vi "hse-application_SetApplicationVersion.vi"(8 "error in":errorcluster, 10 "Application Version History":string, 11 "Application Version Number":string) -> (0 "error out":errorcluster)   [LabVIEW 2014, in "hse-application.lvclass"]
doc: "Stores the version number of the application for later usage (display, logging, ...).\n\n\n\n____\nHAMPEL SOFTWARE ENGINEERING v0.12.0 (2018-09-13 18:21)"
uses:
  hse-application.lvclass
  hse-application.lvclass/hse-application.ctl
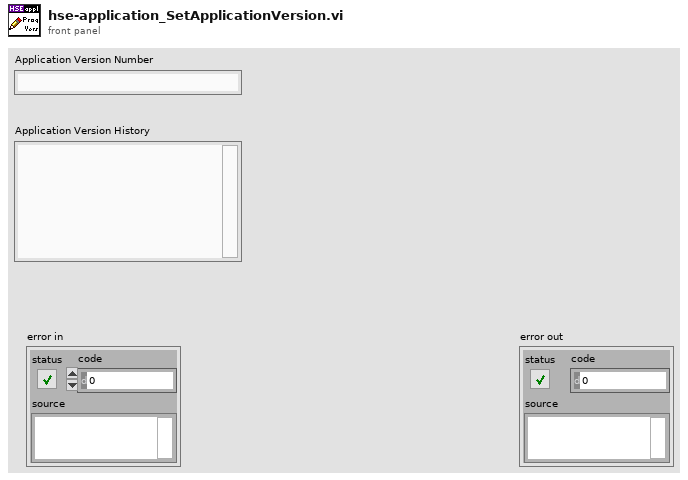
[diagram p1: front panel]
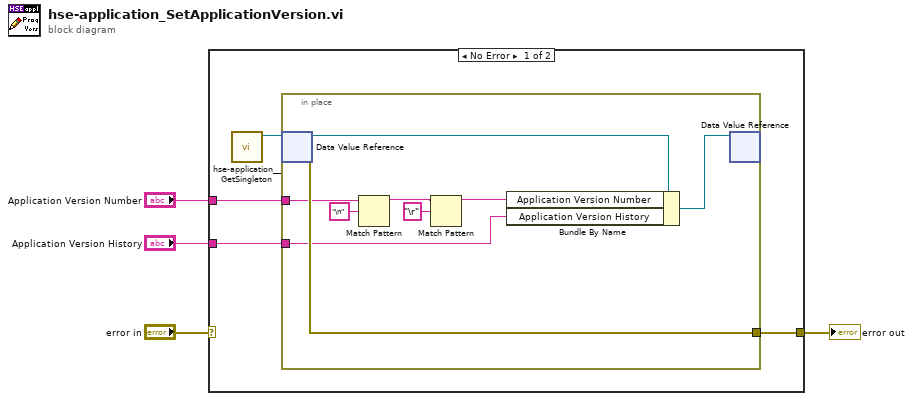
[diagram p0: block diagram]
diagram:
  n1 = case shown="No Error" "error in" {
    selector: "error in" -> [_ w18]
    tunnel: [w7 w18] -> w3
    tunnel: "Application Version Number" -> [w6 _]
    tunnel: "Application Version History" -> [w5 _]
    frame No Error {
      n2 = call "hse-application__GetSingleton.vi"() -> ("ApplicationClass DVR"=w8:refnum<data-value>)  [unwired: 10 in, 1 out]
      n3 = in-place {
        in-place-border: [w17] -> w7
        in-place-border: w6 -> [w14]
        in-place-border: w5 -> [w13]
        n4 = in-place-dvr #1(w8) -> (w16:refnum<class "hse-application.lvclass">, w17:errorcluster)
        n5 = Match Pattern(string=w14, regular expression="\n") -> (before substring=w10:string)  [unwired: 1 in, 3 out]
        n6 = Match Pattern(string=w10, regular expression="\r") -> (before substring=w9:string)  [unwired: 1 in, 3 out]
        n7 = Bundle By Name(cluster=w16, "Application Version Number"=w9, "Application Version History"=w13) -> (w12:refnum<class "hse-application.lvclass">)
        n8 = in-place-dvr #1(w12) -> ()  [unwired: 2 out]
      }
    }
    frame Error {
    }
  }
  "error out" <- w3
